vi "8 and 4 pulses TX 8spc_ver2.vi"(7 "reset system clock":bool, 8 "referenses":T1={"clock x2"="IO Socket\\Data Clock 2x", "Memory In"="pulse on memory", "Memory In 2"="pulse on memory", "Memory In 3"="pulse on memory", "Memory In 4"="pulse on memory"}, 9 "IQ_run":bool=TRUE, 10 "PDW input Valid":bool, 11 "array PDW":u64[](array[numeric])=[0, 0, 0, 0]) -> (0 "trig out":bool, 1 "pulse TX status":T2, 2 "output valid":bool, 3 "IQ out":T3[](array[typedef]), 4 "ready for input":bool)   [LabVIEW 2021]
uses:
  <instrlib>/_niInstr/DSP/v1/Shared/Public/IQ Data.ctl
  pulse_tx_vis/CTL/mode_type.ctl
  <instrlib>/_niInstr/Basic Elements/v1/FPGA/Private/Count Up U64.vi
  <instrlib>/_niInstr/Basic Elements/v1/FPGA/Private/Count Up U32.vi
  <instrlib>/_niInstr/Basic Elements/v1/FPGA/niInstr Basic Elements v1 FPGA.lvlib
  <instrlib>/_niInstr/DSP/v1/Shared/niInstr DSP v1 Shared.lvlib
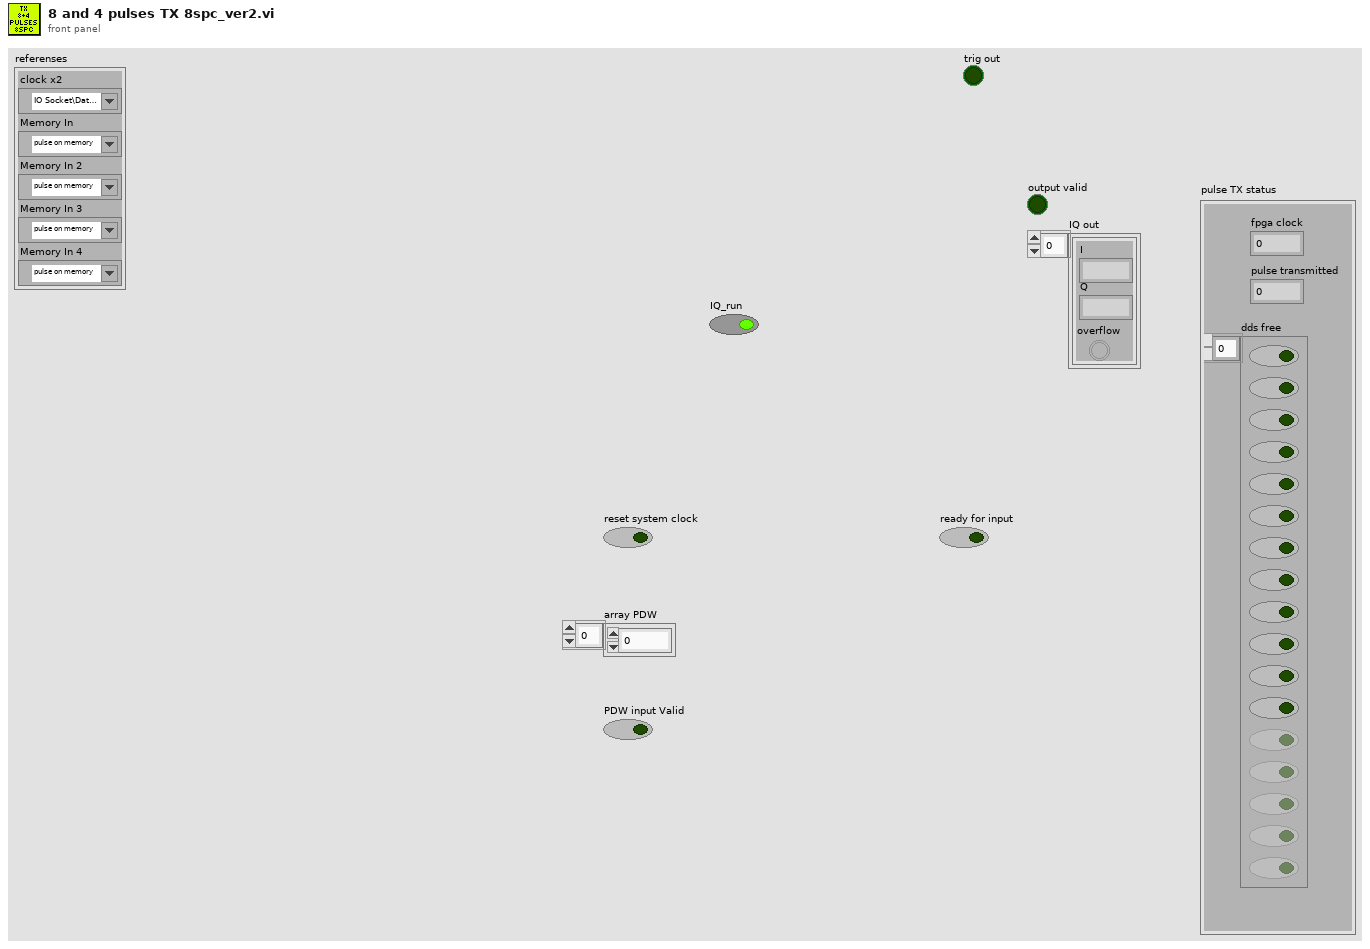
[diagram p1: front panel]
types:
  T1 = cluster{"clock x2":refnum<k21>, "Memory In":refnum<k21>, "Memory In 2":refnum<k21>, "Memory In 3":refnum<k21>, "Memory In 4":refnum<k21>}
  T2 = cluster{"fpga clock":u64, "pulse transmitted":u32, "dds free":bool[]}
  T3 = typedef "niInstr DSP v1 Shared.lvlib/IQ Data.ctl" = cluster{"I":fxp<+/-,18,1>, "Q":fxp<+/-,18,1>, "overflow":bool}
  T4 = typedef "mode_type.ctl" = enum8{"CW", "from memory 1", "NC - cw", "LFM", "BPSK", "QPSK"}
  T5 = typedef "pdw.ctl" = cluster{"PW":u32, "frequency shift":fxp<+/-,48,0>, "amp":fxp<+/-,18,1>, "mode type":T4, "mode depth":u32, "mode filter":u8, "phase shift":fxp<+/-,16,1>, "pulse shape filter":u8}
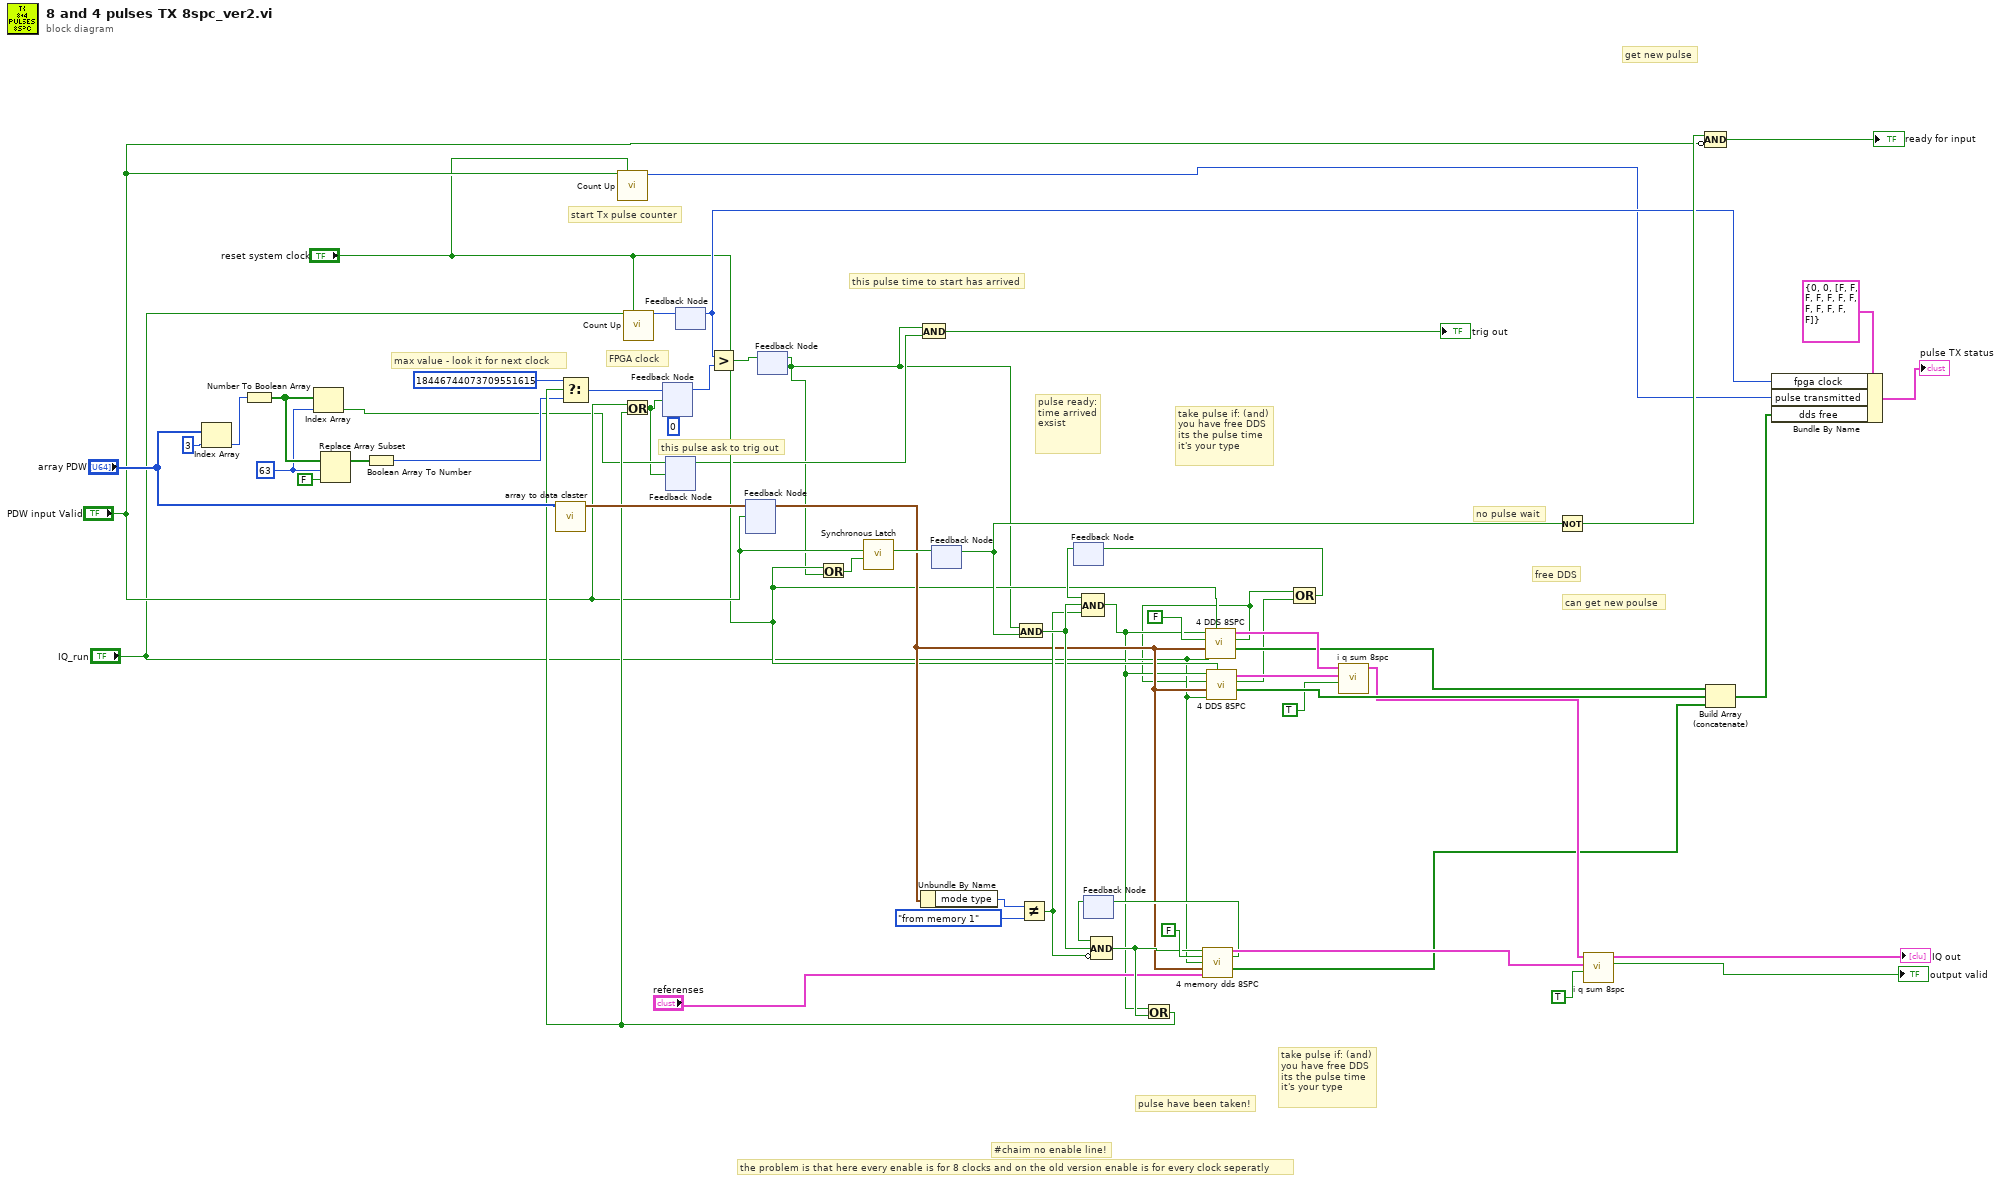
[diagram p0: block diagram]
diagram:
  w10 = 63 ("index")
  # "this pulse ask to trig out"
  # "pulse ready:\ntime arrived\nexsist"
  # "take pulse if: (and)\nyou have free DDS\nits the pulse time\nit's your type"
  # "take pulse if: (and)\nyou have free DDS\nits the pulse time\nit's your type"
  # "pulse have been taken!"
  # "the problem is that here every enable is for 8 clocks and on the old version enable is for every clock seperatly"
  # "#chaim no enable line!"
  # "start Tx pulse counter"
  # "FPGA clock"
  # "this pulse time to start has arrived"
  # "max value - look it for next clock"
  # "get new pulse"
  # "can get new poulse"
  # "no pulse wait"
  # "free DDS"
  n1 = Index Array(array="array PDW", index=3) -> (element=w12:u64)
  n2 = Number To Boolean Array(number=w12) -> (Boolean array=w11:bool[])
  n3 = Index Array(array=w11, index=w10) -> (element=w6:bool)
  n4 = Replace Array Subset(array=w11, new element=FALSE ("new element/subarray"), index=w10) -> (w8:bool[])
  n5 = Boolean Array To Number(Boolean array=w8) -> (number=w7:u64)
  n6 = call "array to data claster.vi"("Array"="array PDW") -> ("Cluster"=w43:T5)  [unwired: 10 in]
  n7 = call-poly <instrlib>:"Count Up.vi"("increment"="PDW input Valid", "reset"="reset system clock") -> ("count out"=w47:u32)  [unwired: 13 in]
  n8 = call-poly <instrlib>:"Count Up.vi"("increment"="IQ_run", "reset"="reset system clock") -> ("count out"=w57:u64)  [unwired: 13 in]
  n9 = feedback #1(u64 0 ("U64")) -> (w51:u64)
  n10 = feedback #2() -> (w4:bool)  [unwired: 1 in]
  n11 = feedback #3() -> (w48:u64)  [unwired: 1 in]
  n12 = feedback-in #3(w57) -> ()
  n13 = Greater?(x=w48, y=w51) -> (0:w61:bool)
  n14 = feedback #4() -> (w19:T5)  [unwired: 1 in]
  n15 = feedback-in #4(w43, "PDW input Valid") -> ()
  n16 = feedback #5() -> (w3:bool)  [unwired: 1 in]
  n17 = feedback-in #5(w61) -> ()
  n18 = Or(x="reset system clock", y=w3) -> (x .or. y?=w24:bool)
  n19 = call <instrlib>:"Synchronous Latch.vi"("clear"=w24, "set"="PDW input Valid") -> ("out"=w22:bool)  [unwired: 9 in]
  n20 = And(x=w3, y=w4) -> (x .and. y?=→"trig out":bool)
  n21 = Unbundle By Name(w19) -> ("mode type"=w45:T4)
  n22 = feedback #6() -> (w21:bool)  [unwired: 1 in]
  n23 = feedback-in #6(w22) -> ()
  n24 = And(x=w3, y=w21) -> (x .and. y?=w40:bool)
  n25 = Not Equal?(x=w45, y=mode_type."from memory 1") -> (x != y?=w39:bool)
  n26 = feedback #7() -> (w30:bool)  [unwired: 1 in]
  n27 = Compound Arithmetic op=AND(w30, w40, w39) -> (w17:bool)
  n28 = feedback #8() -> (w34:bool)  [unwired: 1 in]
  n29 = Compound Arithmetic op=AND(w34, w40, invert w39) -> (w33:bool)
  n30 = Or(x=w17, y=w33) -> (x .or. y?=w32:bool)
  n31 = Select(t=u64 18446744073709551615, s=w32, f=w7) -> (s? t:f=w55:u64)
  n32 = Or(x="PDW input Valid", y=w32) -> (x .or. y?=w5:bool)
  n33 = feedback-in #1(w55, w5) -> ()
  n34 = feedback-in #2(w6, w5) -> ()
  n35 = call "4 memory dds 8SPC.vi"("new PDW in"=w33, "free DDS before me?"=FALSE, "run"="IQ_run", "pdw in"=w19, "referenses"="referenses") -> ("IQ out"=w36:T3[], "have free DDS"=w35:bool, "state of every DDS"=w1:bool[])  [unwired: 7 in, 1 out]
  n36 = feedback-in #8(w35) -> ()
  n37 = call "4 DDS 8SPC.vi"("clear DDS"="reset system clock", "input valid"="IQ_run", "pdw in"=w19, "free DDS before me?"=FALSE, "new PDW in"=w17) -> ("state of every DDS"=w26:bool[], "have free DDS"=w15:bool, "IQ out"=w29:T3[])  [unwired: 3 in, 1 out]
  n38 = call "4 DDS 8SPC.vi"("clear DDS"="reset system clock", "input valid"="IQ_run", "pdw in"=w19, "free DDS before me?"=w15, "new PDW in"=w17) -> ("state of every DDS"=w25:bool[], "have free DDS"=w14:bool, "IQ out"=w28:T3[])  [unwired: 3 in, 1 out]
  n39 = Compound Arithmetic op=OR(w15, w14) -> (w27:bool)
  n40 = feedback-in #7(w27) -> ()
  n41 = call "i q sum 8spc.vi"("input valid"=TRUE, "IQ in 2"=w28, "IQ in"=w29) -> ("IQ out"=w20:T3[])  [unwired: 7 in, 1 out]
  n42 = Not(x=w21) -> (.not. x?=w52:bool)
  n43 = call "i q sum 8spc.vi"("input valid"=TRUE, "IQ in 2"=w36, "IQ in"=w20) -> ("output valid"=→"output valid":bool, "IQ out"=→"IQ out":T3[])  [unwired: 7 in]
  n44 = Compound Arithmetic op=AND(w52, invert "PDW input Valid") -> (→"ready for input":bool)
  n45 = Build Array (concatenate)(w26, w25, w1) -> (w46:bool[])
  n46 = Bundle By Name(cluster=T2 {"fpga clock"=0, "pulse transmitted"=0, "dds free"=[FALSE, FALSE, FALSE, FALSE, FALSE, FALSE, FALSE, FALSE, FALSE, FALSE, FALSE, FALSE]} ("pulse TX status"), "fpga clock"=w48, "pulse transmitted"=w47, "dds free"=w46) -> (→"pulse TX status":T2)
